vi "selection.tester.vi"() -> ()   [LabVIEW 2024]
uses:
  selection_dropdown/Typedefs/Selection Dropdown--cluster.ctl
  selection_dropdown/selection_dropdown.lvclass
  comic_manager/manager_daemon/type_defs/sub-map--map.ctl
  comic_manager/manager_daemon/type_defs/SubData--cluster.ctl
  <vilib>/addons/_JKI Toolkits/State Machine/_JKI_lib_State_Machine.llb/Select State(s)_err__jki_lib_state_machine.vi
  <vilib>/addons/_JKI Toolkits/State Machine/_JKI_lib_State_Machine.llb/Periodic Trigger__ogtk__JKI-SM__jki_lib_state_machine.vi
  comic_manager/manager_daemon/manager_daemon.lvclass
panel:
  in  "Path":path=path "D:/comics/data/key_maps/chars.bin"
  in  "Exit":bool
  in  "selection dropdown":T1
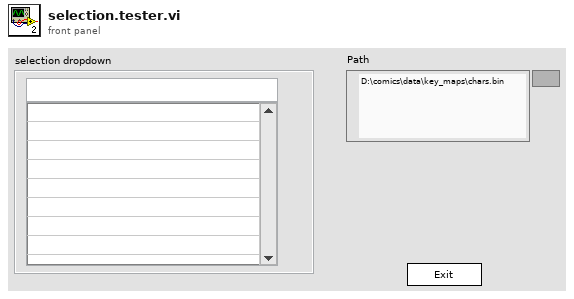
[diagram p1: front panel]
types:
  T1 = typedef "selection_dropdown.lvclass/Selection Dropdown--cluster.ctl" = cluster{"delete":bool, "available":i32, "list":i32, "cancel":bool, "selection":string, "delete all":bool}
  T2 = enum32{"Invalid", "Standard", "Closed", "Hidden", "Minimized", "Maximized"}
  T3 = enum32{"invalid app kind", "Development System", "Run Time System", "Student Edition", "Embedded LabVIEW", "Evaluation", "Custom"}
  T4 = typedef "manager_daemon.lvclass/sub-map--map.ctl" = map{string, T5}
  T5 = typedef "manager_daemon.lvclass/SubData--cluster.ctl" = cluster{"id":i32, "issues":set{i32}}
  T6 = cluster{"Core":cluster{"Current VI Reference":refnum<vi>, "Close Panel on Exit?":bool}, "selection class":refnum<class "selection_dropdown.lvclass">}
  T7 = cluster{"Current VI Reference":refnum<vi>, "Close Panel on Exit?":bool}
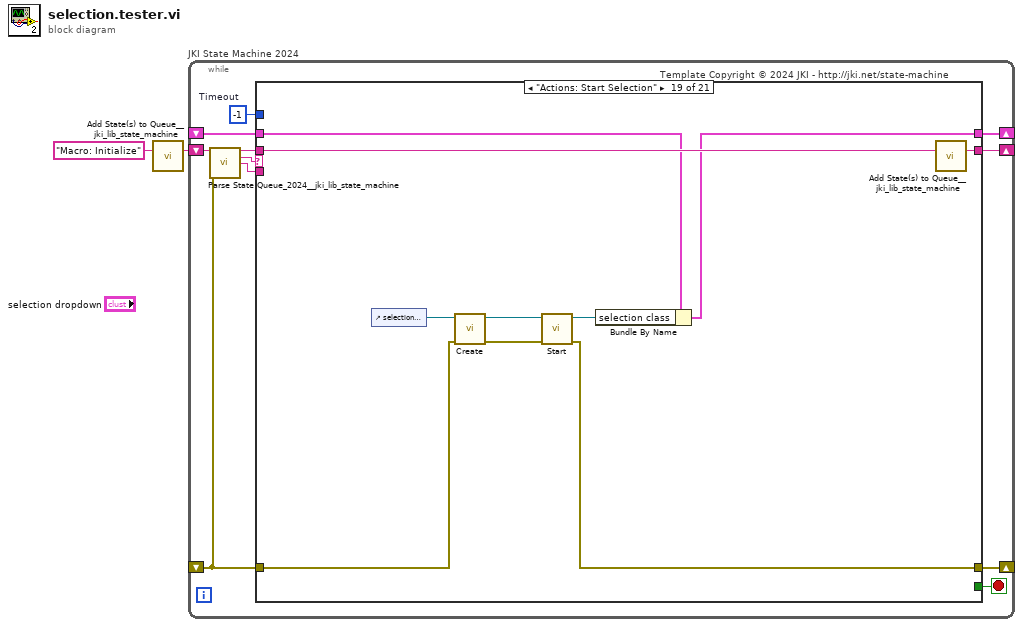
[diagram p0: block diagram]
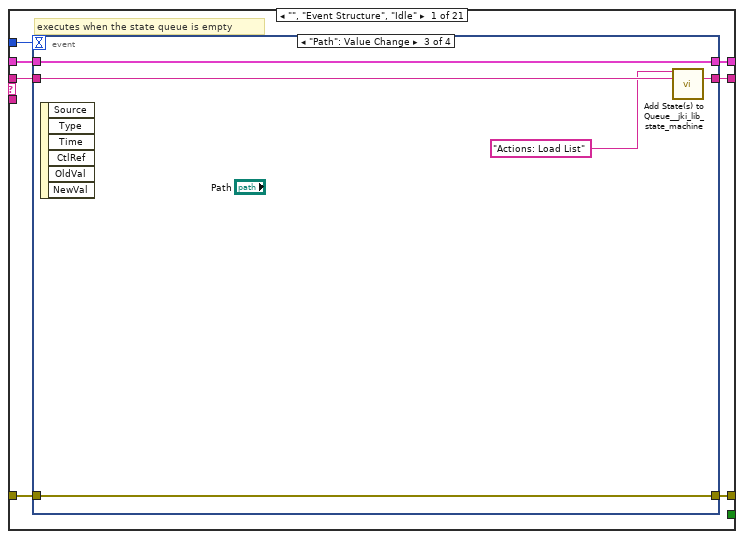
[diagram p2: hidden frame]
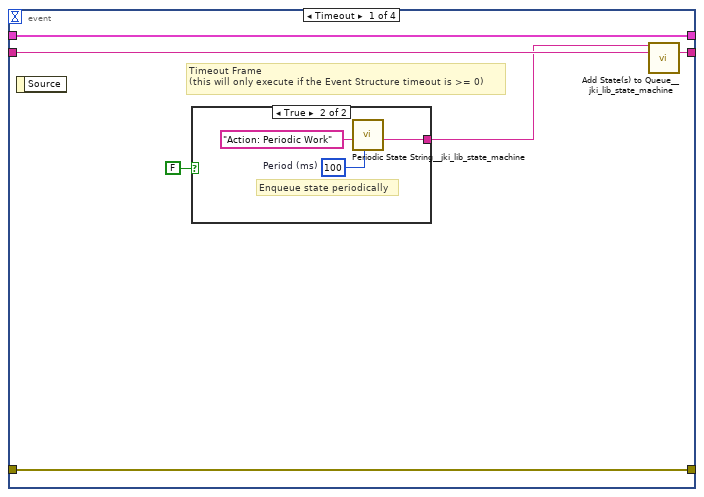
[diagram p3: hidden frame]
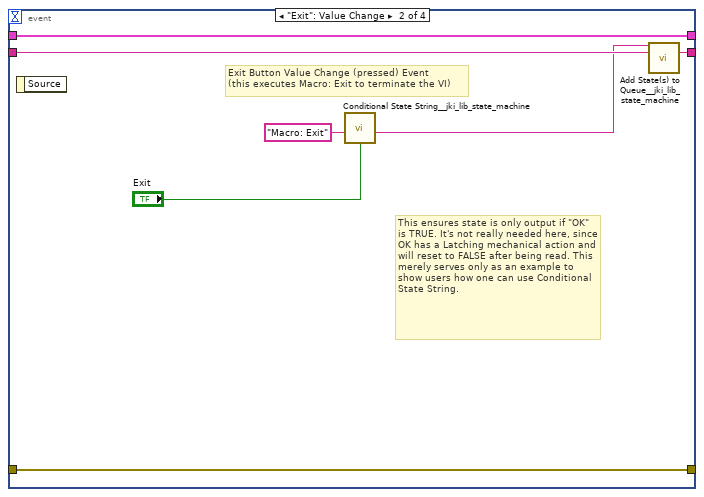
[diagram p5: hidden frame]
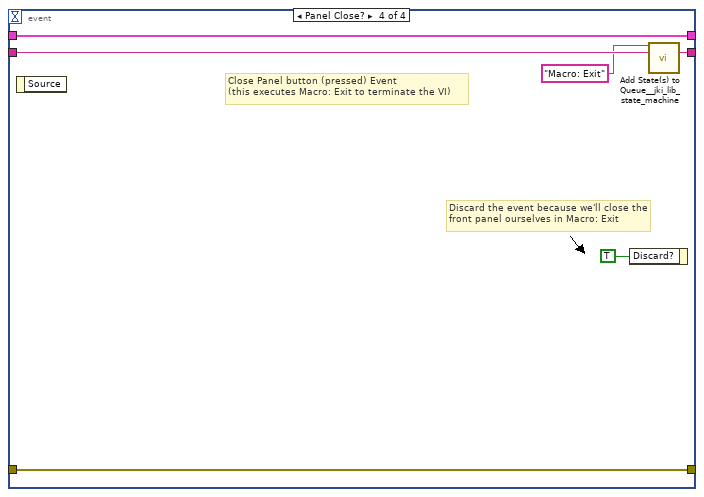
[diagram p6: hidden frame]
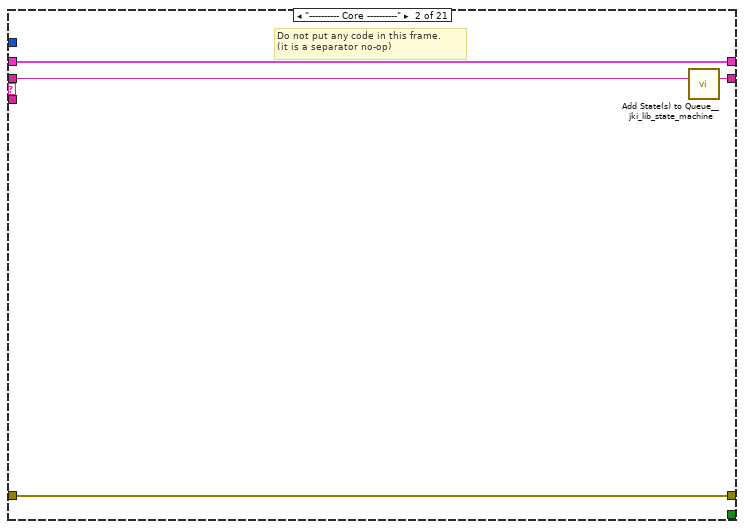
[diagram p7: hidden frame]
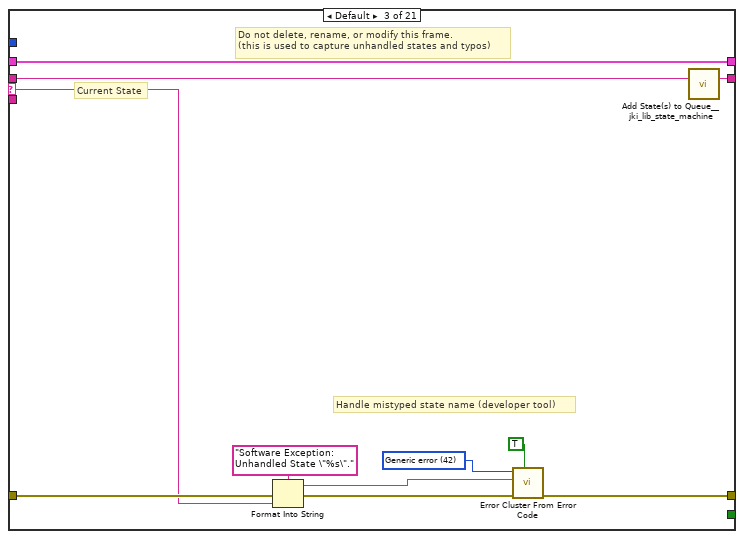
[diagram p8: hidden frame]
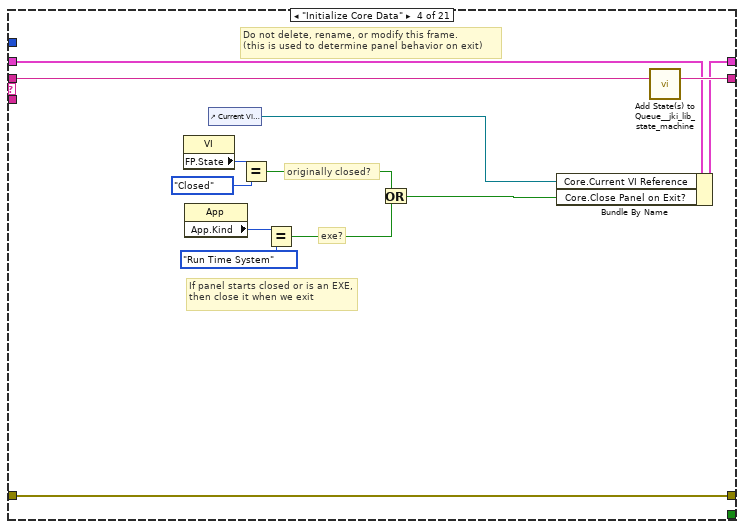
[diagram p9: hidden frame]
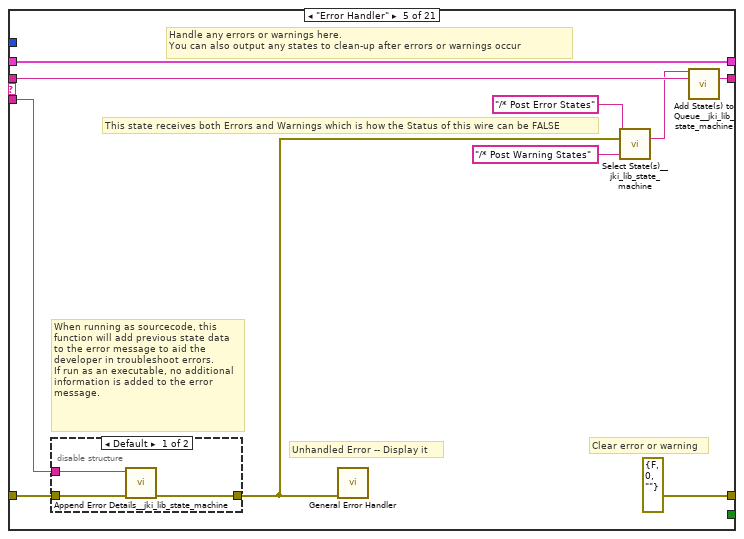
[diagram p10: hidden frame]
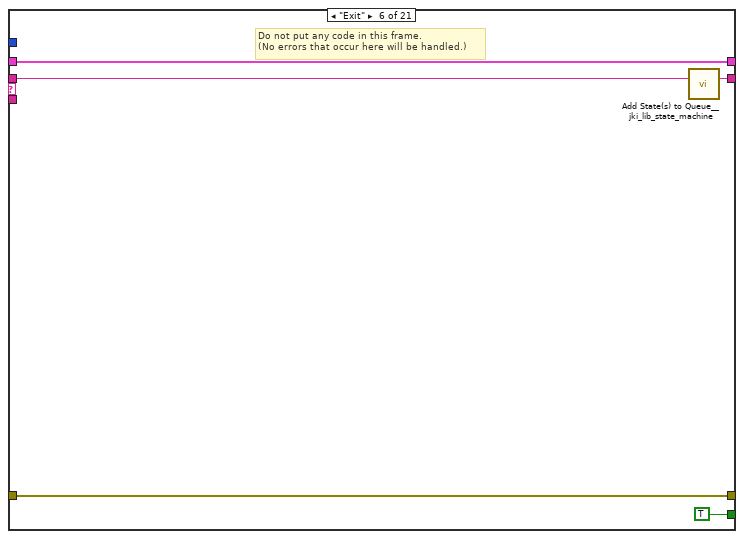
[diagram p12: hidden frame]
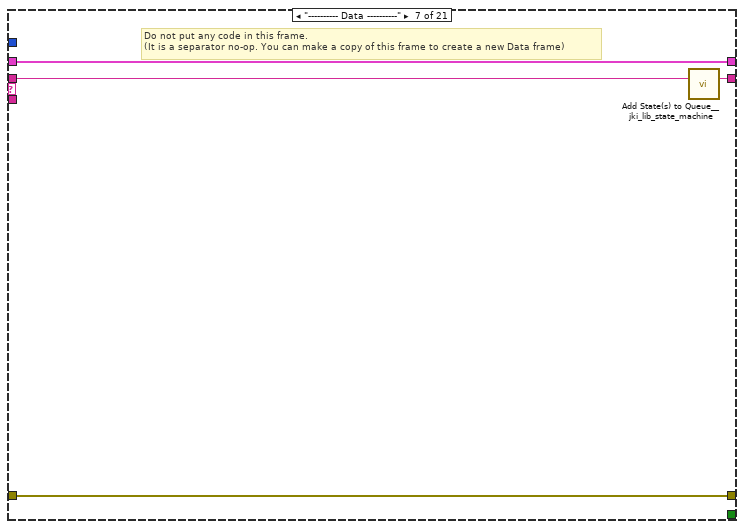
[diagram p13: hidden frame]
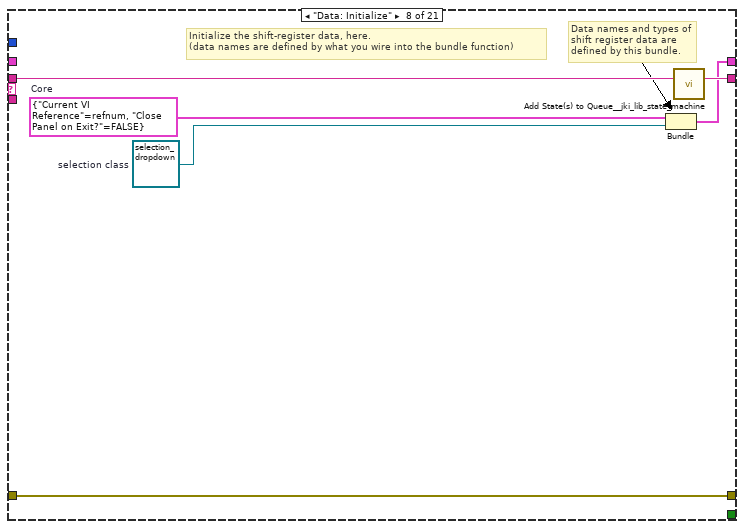
[diagram p14: hidden frame]
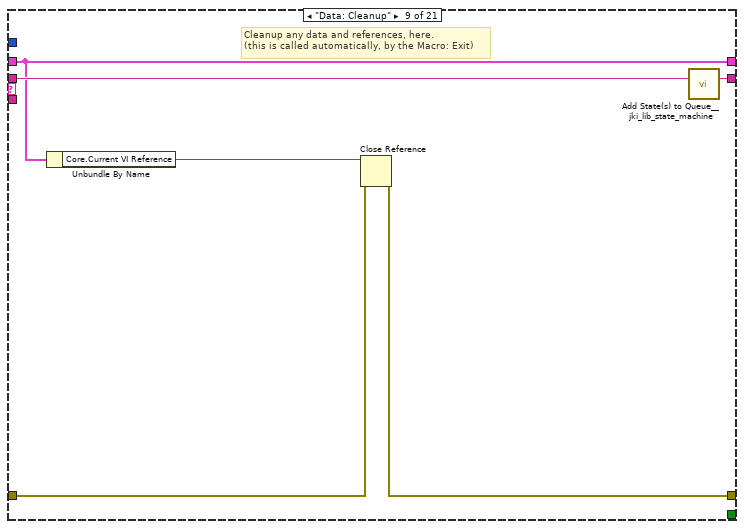
[diagram p15: hidden frame]
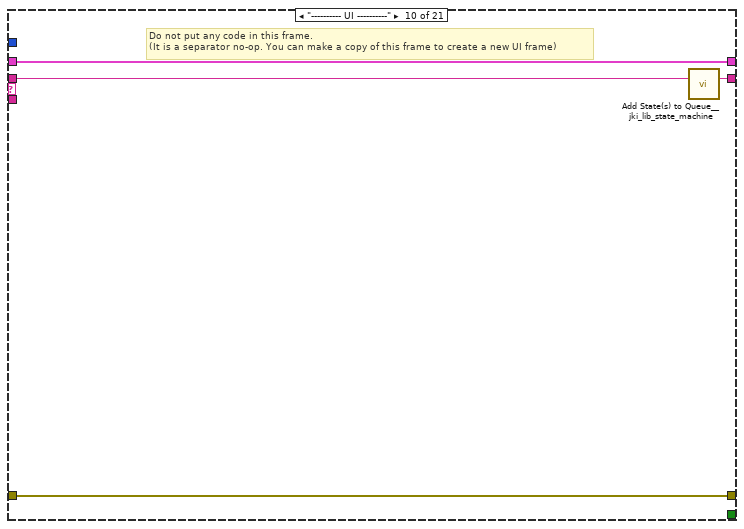
[diagram p16: hidden frame]
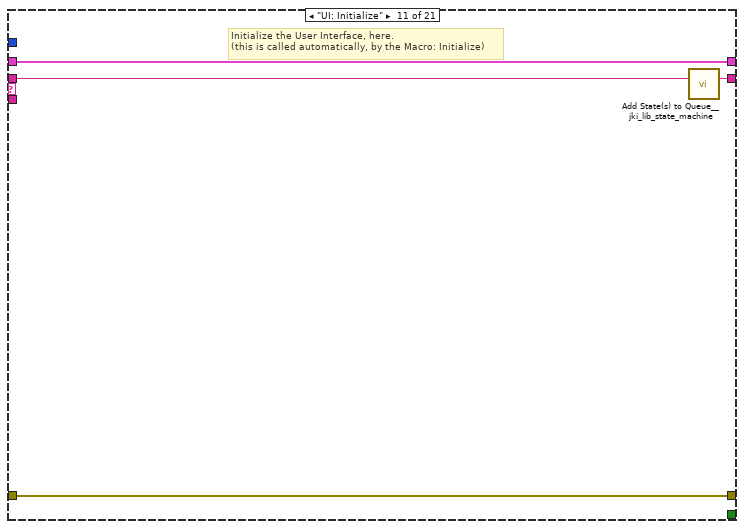
[diagram p17: hidden frame]
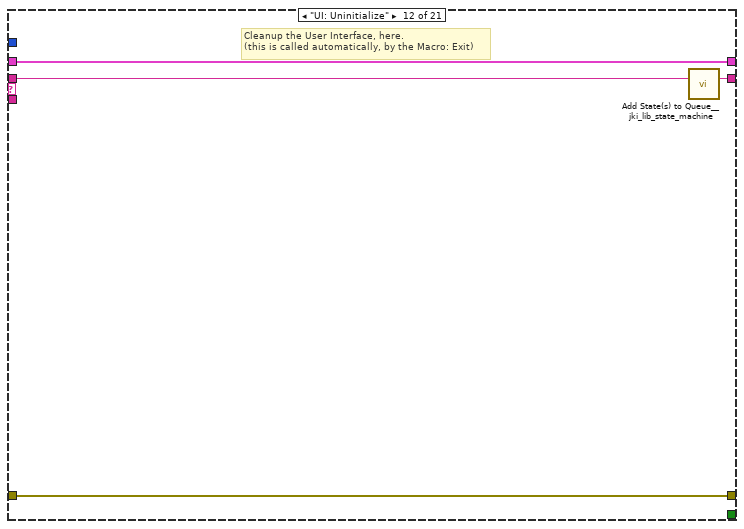
[diagram p18: hidden frame]
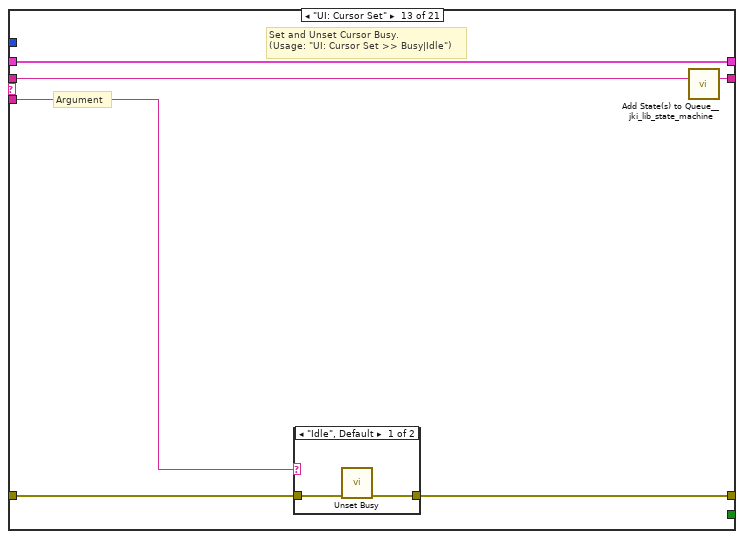
[diagram p19: hidden frame]
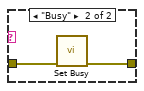
[diagram p20: hidden frame]
diagram:
  n1 = call <vilib>:"Add State(s) to Queue__jki_lib_state_machine.vi"("State(s) in (\"\")"="Macro: Initialize") -> ("States Out"=w2:string)  [unwired: 14 in]
  n2 = while "JKI State Machine 2024" {
    shift-right: [w6] -> _
    shift-left: _ -> [w5]
    shift-right: [w9] -> _
    shift-left: _ -> [w3]
    shift-right: [w8] -> _
    shift-left: w2 -> [w10]
    stop <- w7 stop-if-true
    w4 = -1  # Timeout
    # "Template Copyright © 2024 JKI - http://jki.net/state-machine"
    n3 = call <vilib>:"Parse State Queue_2024__jki_lib_state_machine.vi"("State Queue"=w10, "Error In (no error)"=w3) -> ("Remaining States"=w12:string, "Current State"=w13:string, "Arguments"=w11:string)  [unwired: 11 in]
    n4 = case shown="\"Actions: Start Selection\"" w13 {
      selector: w13 -> [_ _ w52 _ _ _ _ _ _ _ _ _ _ _ _ _ _ _ _ _ _]
      tunnel: w12 -> [w20 w51 w56 w75 w85 w94 w98 w104 w110 w114 w118 w122 w128 w139 w208 w213 w222 w226 w236 w242 w252]
      tunnel: w11 -> [_ _ _ _ w80 _ _ _ _ _ _ _ w123 w133 _ _ _ _ _ _ _]
      tunnel: w5 -> [w18 w48 w54 w68 w82 w92 w95 _ w105 w111 w116 w120 w126 w135 w205 w210 w220 w223 w230 w240 w250]
      tunnel: [w17 w49 w58 w72 errorcluster {"status"=FALSE, "code"=0, "source"=""} ("error out") w91 w96 w101 w106 w112 w115 w119 w124 w136 w206 w211 w217 w224 w231 w237 w248] -> w9
      tunnel: w3 -> [w14 w49 w57 w72 w81 w91 w96 w101 w107 w112 w115 w119 w125 w137 w206 w211 w217 w224 w234 w238 w247]
      tunnel: [w19 w50 w55 w74 w84 w93 w97 w103 w109 w113 w117 w121 w127 w138 w207 w212 w221 w225 w235 w241 w251] -> w8
      tunnel: [_ _ _ _ _ TRUE _ _ _ _ _ _ _ _ _ _ _ _ _ _ _] -> w7
      tunnel: [w16 w48 w54 w73 w82 w92 w95 w102 w105 w111 w116 w120 w126 w135 w205 w210 w220 w223 w229 w240 w250] -> w6
      tunnel: w4 -> [w15 _ _ _ _ _ _ _ _ _ _ _ _ _ _ _ _ _ _ _ _]
      frame "", "Event Structure", "Idle" {
        # "executes when the state queue is empty"
        n5 = event shown="[2] \"Path\": Value Change" {
          selector: _ -> [_ _ _ _]
          dyn-events: _ -> [_ _ _ _]
          timeout: w15 -> [_ _ _ _]
          tunnel: w20 -> [w26 w36 w41 w47]
          tunnel: [w25 w35 w40 w46] -> w19
          tunnel: w18 -> [w23 w33 w38 w44]
          tunnel: [w24 w34 w39 w45] -> w17
          tunnel: w14 -> [w24 w34 w39 w45]
          tunnel: [w23 w33 w38 w44] -> w16
          event Timeout {
            # "Timeout Frame\n(this will only execute if the Event Structure timeout is >= 0)"
            n6 = event-data() -> ()  [unwired: 1 in, 1 out]
            n7 = case shown="True" FALSE {
              tunnel: [_ w29] -> w22
              frame False {
              }
              frame True {
                w27 = u32 100  # Period (ms)
                # "Enqueue state periodically"
                n8 = call <vilib>:"Periodic State String__jki_lib_state_machine.vi"("Period (ms)"=w27, "State"="Action: Periodic Work") -> ("State Out"=w29:string)  [unwired: 9 in]
              }
            }
            n9 = call <vilib>:"Add State(s) to Queue__jki_lib_state_machine.vi"("State(s) in Front (\"\")"=w22, "State(s) in (\"\")"=w26) -> ("States Out"=w25:string)  [unwired: 13 in]
          }
          event "Exit": Value Change {
            # "This ensures state is only output if \"OK\" is TRUE. It's not really needed here, since OK has a Latching mechanical action and will reset to FALSE after being read. This merely serves only as an example to show users how one can use Conditional State String."
            # "Exit Button Value Change (pressed) Event\n(this executes Macro: Exit to terminate the VI)"
            n10 = event-data() -> ()  [unwired: 1 in, 1 out]
            n11 = call <vilib>:"Conditional State String__jki_lib_state_machine.vi"("Do State(s)?"="Exit", "State"="Macro: Exit") -> ("State Out"=w30:string)  [unwired: 7 in]
            n12 = call <vilib>:"Add State(s) to Queue__jki_lib_state_machine.vi"("State(s) in Front (\"\")"=w30, "State(s) in (\"\")"=w36) -> ("States Out"=w35:string)  [unwired: 13 in]
          }
          event "Path": Value Change {
            n13 = event-data() -> ()  [unwired: 1 in, 6 out]
            n14 = call <vilib>:"Add State(s) to Queue__jki_lib_state_machine.vi"("State(s) in Front (\"\")"="Actions: Load List", "State(s) in (\"\")"=w41) -> ("States Out"=w40:string)  [unwired: 13 in]
          }
          event Panel Close? {
            # "Discard the event because we'll close the front panel ourselves in Macro: Exit"
            # "Close Panel button (pressed) Event\n(this executes Macro: Exit to terminate the VI)"
            n15 = event-data() -> ()  [unwired: 1 in, 1 out]
            n16 = event-data("Discard?"=TRUE) -> ()  [unwired: 1 in, 1 out]
            n17 = call <vilib>:"Add State(s) to Queue__jki_lib_state_machine.vi"("State(s) in Front (\"\")"="Macro: Exit", "State(s) in (\"\")"=w47) -> ("States Out"=w46:string)  [unwired: 13 in]
          }
        }
      }
      frame "---------- Core ----------" {
        # "Do not put any code in this frame.\n(it is a separator no-op)"
        n18 = call <vilib>:"Add State(s) to Queue__jki_lib_state_machine.vi"("State(s) in (\"\")"=w51) -> ("States Out"=w50:string)  [unwired: 14 in]
      }
      frame Default {
        w61 = 42 items=["No error", "Argument error", "Memory is full", "Out of zone", "End of file", "File already open", "Generic file I/O error", "File not found", "File permission error", "Disk is full", "Duplicate path", "Too many files open", "System feature not enabled", "Resource file not found", "Cannot add resource", "Resource not found", "Image not found", "Image memory error", "Pen does not exist", "Config type invalid", "Config token not found", "Config parse error", "Config memory error", "Bad external code format", "Bad external code offset", "External code not present", "Null window", "Destroy window error", "Null menu", "Print aborted", "Bad print record", "Print driver error", "Windows error during printing", "Memory error during printing", "Print dialog error", "Generic print error", "Invalid device refnum", "Device not found", "Device parameter error", "Device unit error", "Cannot open device", "Device call aborted", "Generic error", "Cancelled by user", "Object ID too low", "Object ID too high", "Object not in heap", "Unknown heap", "Unknown object (invalid DefProc)", "Unknown object (DefProc not in table)", "Message out of range", "Invalid (null) method", "Unknown message", "Manager call not supported", "Bad address", "Network operation in progress", "Network operation timed out", "Connection is busy", "Network attribute not supported", "Network error", "Address in use", "System out of memory", "Connection aborted", "Connection refused", "Not connected", "Already connected", "Connection closed", "Initialization error (interapplication manager)", "Bad occurrence", "Wait on unbound occurrence handler", "Occurrence queue overflow", "Datalog type conflict", "Unused", "Unrecognized type (interapplication manager)", "Memory corrupt", "Failed to make temporary DLL", "Old CIN version", "Drag socket not found", "Failed to load drop-object", "Failed to register OLE object", "Failed to release OLE object", "Format specifier type mismatch", "Unknown format specifier", "Too few format specifiers", "Too many format specifiers", "Scan failed", "Newer CIN version", "Error converting to variant", "Runtime menu error", "Password tampered", "Variant attribute not found", "Incompatible variant data type", "Event data is not available", "Event Store is not present", "Occurrence is not found", "Event Queue is not created", "Event info is not available", "Refnum passed is NULL", "Error retrieving Class GUID", "Error retrieving CoClass GUID", "Error retrieving TypeLib GUID.", "Bad built application magic bytes.", "Specific driver is different from the specific driver associated with the Logical Name.", "There is no session opened to the class driver.", "Max Error", "MAX - Error with config objects", "MAX - Error loading configuration", "MAX - Group not supported"]
        # "Current State"
        # "Do not delete, rename, or modify this frame.\n(this is used to capture unhandled states and typos)"
        # "Handle mistyped state name (developer tool)"
        n19 = Format Into String(format string="Software Exception: Unhandled State \"%s\"." ("message"), error in=w57, w52) -> (resulting string=w60:string, error out=w59:errorcluster)  [unwired: 1 in]
        n20 = call <vilib>:"Error Cluster From Error Code.vi"("show call chain? (False)"=TRUE, "error in (no error)"=w59, "error message (\"\")"=w60, "error code (0)"=w61) -> ("error out"=w58:errorcluster)  [unwired: 5 in]
        n21 = call <vilib>:"Add State(s) to Queue__jki_lib_state_machine.vi"("State(s) in (\"\")"=w56) -> ("States Out"=w55:string)  [unwired: 14 in]
      }
      frame "Initialize Core Data" {
        # "Do not delete, rename, or modify this frame.\n(this is used to determine panel behavior on exit)"
        # "originally closed?"
        # "exe?"
        # "If panel starts closed or is an EXE, then close it when we exit"
        n22 = property class="VI"() -> ("FP.State"=w65:T2)  [unwired: 2 in, 2 out]
        n23 = property class="App"() -> ("App.Kind"=w71:T3)  [unwired: 2 in, 2 out]
        n24 = control-ref of="Current VI Reference"() -> (w66:refnum<vi>)
        n25 = Equal?(x=w65, y=T2."Closed" ("Front Panel Window:State")) -> (x = y?=w63:bool)
        n26 = Equal?(x=w71, y=T3."Run Time System" ("Application:Kind")) -> (x = y?=w69:bool)
        n27 = Or(x=w63, y=w69) -> (x .or. y?=w67:bool)
        n28 = Bundle By Name(cluster=w68, "Core.Current VI Reference"=w66, "Core.Close Panel on Exit?"=w67) -> (w73:T6)
        n29 = call <vilib>:"Add State(s) to Queue__jki_lib_state_machine.vi"("State(s) in (\"\")"=w75) -> ("States Out"=w74:string)  [unwired: 14 in]
      }
      frame "Error Handler" {
        # "When running as sourcecode, this function will add previous state data to the error message to aid the developer in troubleshoot errors.\nIf run as an executable, no additional information is added to the error message."
        # "This state receives both Errors and Warnings which is how the Status of this wire can be FALSE"
        # "Unhandled Error -- Display it"
        # "Handle any errors or warnings here.\nYou can also output any states to clean-up after errors or warnings occur"
        # "Clear error or warning"
        n30 = disable-structure shown="Default" {
          disable-tunnel: w81 -> [w88 w89]
          disable-tunnel: w80 -> [w87 _]
          disable-tunnel: [w86 w89] -> w79
          frame condition #0 (active) {
            n31 = call <vilib>:"Append Error Details__jki_lib_state_machine.vi"("error in (no error)"=w88, "Previous State and Argument(s)"=w87) -> ("error out"=w86:errorcluster)  [unwired: 9 in]
          }
          frame condition #1 {
          }
        }
        n32 = call <vilib>:"General Error Handler.vi"("error in (no error)"=w79) -> ()  [unwired: 10 in, 5 out]
        n33 = call-poly <vilib>:"Select State(s)__jki_lib_state_machine.vi"("State(s) if True (\"\")"="/* Post Error States", "Select"=w79, "State(s) if False (\"\")"="/* Post Warning States") -> ("States Out"=w77:string)  [unwired: 12 in]
        n34 = call <vilib>:"Add State(s) to Queue__jki_lib_state_machine.vi"("State(s) in Front (\"\")"=w77, "State(s) in (\"\")"=w85) -> ("States Out"=w84:string)  [unwired: 13 in]
      }
      frame "Exit" {
        # "Do not put any code in this frame.\n(No errors that occur here will be handled.)"
        n35 = call <vilib>:"Add State(s) to Queue__jki_lib_state_machine.vi"("State(s) in (\"\")"=w94) -> ("States Out"=w93:string)  [unwired: 14 in]
      }
      frame "---------- Data ----------" {
        # "Do not put any code in this frame.\n(It is a separator no-op. You can make a copy of this frame to create a new Data frame)"
        n36 = call <vilib>:"Add State(s) to Queue__jki_lib_state_machine.vi"("State(s) in (\"\")"=w98) -> ("States Out"=w97:string)  [unwired: 14 in]
      }
      frame "Data: Initialize" {
        w99 = refnum<class "selection_dropdown.lvclass"> refnum  # selection class
        w100 = T7 {"Current VI Reference"=refnum, "Close Panel on Exit?"=FALSE}  # Core
        # "Data names and types of shift register data are defined by this bundle."
        # "Initialize the shift-register data, here.\n(data names are defined by what you wire into the bundle function)"
        n37 = Bundle("Core"=w100, "selection class"=w99) -> (w102:T6)  [unwired: 1 in]
        n38 = call <vilib>:"Add State(s) to Queue__jki_lib_state_machine.vi"("State(s) in (\"\")"=w104) -> ("States Out"=w103:string)  [unwired: 14 in]
      }
      frame "Data: Cleanup" {
        # "Cleanup any data and references, here.\n(this is called automatically, by the Macro: Exit)"
        n39 = Unbundle By Name(w105) -> ("Core.Current VI Reference"=w108:refnum<vi>)
        n40 = Close Reference(reference=w108, error in (no error)=w107) -> (error out=w106:errorcluster)
        n41 = call <vilib>:"Add State(s) to Queue__jki_lib_state_machine.vi"("State(s) in (\"\")"=w110) -> ("States Out"=w109:string)  [unwired: 14 in]
      }
      frame "---------- UI ----------" {
        # "Do not put any code in this frame.\n(It is a separator no-op. You can make a copy of this frame to create a new UI frame)"
        n42 = call <vilib>:"Add State(s) to Queue__jki_lib_state_machine.vi"("State(s) in (\"\")"=w114) -> ("States Out"=w113:string)  [unwired: 14 in]
      }
      frame "UI: Initialize" {
        # "Initialize the User Interface, here.\n(this is called automatically, by the Macro: Initialize)"
        n43 = call <vilib>:"Add State(s) to Queue__jki_lib_state_machine.vi"("State(s) in (\"\")"=w118) -> ("States Out"=w117:string)  [unwired: 14 in]
      }
      frame "UI: Uninitialize" {
        # "Cleanup the User Interface, here.\n(this is called automatically, by the Macro: Exit)"
        n44 = call <vilib>:"Add State(s) to Queue__jki_lib_state_machine.vi"("State(s) in (\"\")"=w122) -> ("States Out"=w121:string)  [unwired: 14 in]
      }
      frame "UI: Cursor Set" {
        # "Argument"
        # "Set and Unset Cursor Busy.\n(Usage: \"UI: Cursor Set >> Busy|Idle\")"
        n45 = case shown="\"Idle\", Default" w123 {
          tunnel: w125 -> [w130 w132]
          tunnel: [w129 w131] -> w124
          frame "Idle", Default {
            n46 = call <vilib>:"Unset Busy.vi"("error in (no error)"=w130) -> ("error out"=w129:errorcluster)  [unwired: 10 in]
          }
          frame "Busy" {
            n47 = call <vilib>:"Set Busy.vi"("error in (no error)"=w132) -> ("error out"=w131:errorcluster)  [unwired: 9 in, 1 out]
          }
        }
        n48 = call <vilib>:"Add State(s) to Queue__jki_lib_state_machine.vi"("State(s) in (\"\")"=w128) -> ("States Out"=w127:string)  [unwired: 14 in]
      }
      frame "UI: Front Panel State" {
        # "Argument"
        # "Set Front Panel Open or Closed\n(Usage: \"UI: Front Panel State >> Open|Close\")"
        n49 = Unbundle By Name(w135) -> ("Core.Current VI Reference"=w134:refnum<vi>)
        n50 = case shown="\"Minimize\", \"Minimized\"" w133 {
          tunnel: w137 -> [w145 w160 w171 w184 w197]
          tunnel: [w147 w161 w173 w186 w199] -> w136
          tunnel: w134 -> [w146 w158 w172 w185 w198]
          frame "Open", "Standard", Default {
            w140 = T2."Standard" ("State")
            n51 = property class="VI"(reference=w146, error in=w145) -> (reference out=w143:refnum<vi>, error out=w144:errorcluster, "FP.State"=w142:T2)
            n52 = Not Equal?(x=w142, y=w140) -> (x != y?=w141:bool)
            n53 = case shown="True" w141 {
              tunnel: [w151 w153] -> w147
              tunnel: w144 -> [w150 w153]
              tunnel: w143 -> [w149 _]
              tunnel: w140 -> [w148 _]
              frame True {
                n54 = invoke class="VI" method="FP.Open"(reference=w149, error in=w150, "Activate"=TRUE, "State"=w148) -> (error out=w151:errorcluster)  [unwired: 1 in, 4 out]
              }
              frame False {
              }
            }
          }
          frame "Close", "Closed" {
            n55 = property class="VI"(reference=w158, error in=w160) -> (reference out=w157:refnum<vi>, error out=w159:errorcluster, "FP.State"=w155:T2)
            n56 = Not Equal?(x=w155, y=T2."Closed" ("Front Panel Window:State")) -> (x != y?=w154:bool)
            n57 = case shown="True" w154 {
              tunnel: [w162 w165] -> w161
              tunnel: w159 -> [w162 w164]
              tunnel: w157 -> [_ w163]
              frame False {
              }
              frame True {
                n58 = invoke class="VI" method="FP.Close"(reference=w163, error in=w164) -> (error out=w165:errorcluster)  [unwired: 1 in, 2 out]
              }
            }
          }
          frame "Hidden", "Hide" {
            w166 = T2."Hidden" ("State")
            n59 = property class="VI"(reference=w172, error in=w171) -> (reference out=w169:refnum<vi>, error out=w170:errorcluster, "FP.State"=w168:T2)
            n60 = Not Equal?(x=w168, y=w166) -> (x != y?=w167:bool)
            n61 = case shown="True" w167 {
              tunnel: [w177 w178] -> w173
              tunnel: w170 -> [w176 w178]
              tunnel: w169 -> [w175 _]
              tunnel: w166 -> [w174 _]
              frame True {
                n62 = invoke class="VI" method="FP.Open"(reference=w175, error in=w176, "State"=w174) -> (error out=w177:errorcluster)  [unwired: 2 in, 4 out]
              }
              frame False {
              }
            }
          }
          frame "Minimize", "Minimized" {
            w179 = T2."Minimized" ("State")
            n63 = property class="VI"(reference=w185, error in=w184) -> (reference out=w182:refnum<vi>, error out=w183:errorcluster, "FP.State"=w181:T2)
            n64 = Not Equal?(x=w181, y=w179) -> (x != y?=w180:bool)
            n65 = case shown="True" w180 {
              tunnel: [w190 w191] -> w186
              tunnel: w183 -> [w189 w191]
              tunnel: w182 -> [w188 _]
              tunnel: w179 -> [w187 _]
              frame True {
                n66 = invoke class="VI" method="FP.Open"(reference=w188, error in=w189, "State"=w187) -> (error out=w190:errorcluster)  [unwired: 2 in, 4 out]
              }
              frame False {
              }
            }
          }
          frame "Maximize", "Maximized" {
            w192 = T2."Maximized" ("State")
            n67 = property class="VI"(reference=w198, error in=w197) -> (reference out=w195:refnum<vi>, error out=w196:errorcluster, "FP.State"=w194:T2)
            n68 = Not Equal?(x=w194, y=w192) -> (x != y?=w193:bool)
            n69 = case shown="True" w193 {
              tunnel: [w203 w204] -> w199
              tunnel: w196 -> [w202 w204]
              tunnel: w195 -> [w201 _]
              tunnel: w192 -> [w200 _]
              frame True {
                n70 = invoke class="VI" method="FP.Open"(reference=w201, error in=w202, "State"=w200) -> (error out=w203:errorcluster)  [unwired: 2 in, 4 out]
              }
              frame False {
              }
            }
          }
        }
        n71 = call <vilib>:"Add State(s) to Queue__jki_lib_state_machine.vi"("State(s) in (\"\")"=w139) -> ("States Out"=w138:string)  [unwired: 14 in]
      }
      frame "---------- Macro ----------" {
        # "Do not put any code in this frame.\n(It is a separator no-op. You can make a copy of this frame to create a new Macro frame)"
        n72 = call <vilib>:"Add State(s) to Queue__jki_lib_state_machine.vi"("State(s) in (\"\")"=w208) -> ("States Out"=w207:string)  [unwired: 14 in]
      }
      frame "Macro: Initialize" {
        w209 = "Data: Initialize\nInitialize Core Data\nUI: Initialize\nUI: Front Panel State >> Open\nActions: Start Selection\nActions: Load List"  # Data: Initialize Initialize Core Data UI: Initialize UI: Front Panel State >> Open Actions: Start Selection Actions: Load List
        # "Initialization Macro\n(This is called once, when the VI starts)"
        n73 = call <vilib>:"Add State(s) to Queue__jki_lib_state_machine.vi"("State(s) in Front (\"\")"=w209, "State(s) in (\"\")"=w213) -> ("States Out"=w212:string)  [unwired: 13 in]
      }
      frame "Macro: Exit" {
        # "Exit Macro\n(This is called once, when the VI exits)"
        n74 = Unbundle By Name(w220) -> ("Core.Close Panel on Exit?"=w215:bool)
        n75 = call <vilib>:"Conditional State String__jki_lib_state_machine.vi"("Do State(s)?"=w215, "State"="UI: Front Panel State >> Close") -> ("State Out"=w214:string)  [unwired: 7 in]
        n76 = call <vilib>:"Add State(s) to Queue__jki_lib_state_machine.vi"("State(s) in (\"\")"=w214, "State(s) at Back (\"\")"="UI: Uninitialize\nData: Cleanup\nActions: Close Selection\nExit") -> ("States Out"=w218:string)  [unwired: 13 in]
        n77 = call <vilib>:"Add State(s) to Queue__jki_lib_state_machine.vi"("State(s) in Front (\"\")"=w218, "State(s) in (\"\")"=w222) -> ("States Out"=w221:string)  [unwired: 13 in]
      }
      frame "---------- Actions ----------" {
        # "Template Separator\n(You can make a copy of, or modify, this frame)"
        n78 = call <vilib>:"Add State(s) to Queue__jki_lib_state_machine.vi"("State(s) in (\"\")"=w226) -> ("States Out"=w225:string)  [unwired: 14 in]
      }
      frame "Actions: Start Selection" {
        n79 = control-ref of="selection dropdown"() -> (w227:refnum<vi>)
        n80 = call "Create.vi"("error in (no error)"=w234, "ref"=w227) -> ("error out"=w233:errorcluster, "selection_dropdown out"=w232:refnum<class "selection_dropdown.lvclass">)  [unwired: 8 in]
        n81 = call "Start.vi"("error in (no error)"=w233, "selection_dropdown in"=w232) -> ("error out"=w231:errorcluster, "selection_dropdown out"=w228:refnum<class "selection_dropdown.lvclass">)  [unwired: 8 in]
        n82 = Bundle By Name(cluster=w230, "selection class"=w228) -> (w229:T6)
        n83 = call <vilib>:"Add State(s) to Queue__jki_lib_state_machine.vi"("State(s) in (\"\")"=w236) -> ("States Out"=w235:string)  [unwired: 14 in]
      }
      frame "Actions: Close Selection" {
        n84 = Unbundle By Name(w240) -> ("selection class"=w239:refnum<class "selection_dropdown.lvclass">)
        n85 = call "Destroy.vi"("error in (no error)"=w238, "selection_dropdown in"=w239) -> ("error out"=w237:errorcluster)  [unwired: 8 in, 1 out]
        n86 = call <vilib>:"Add State(s) to Queue__jki_lib_state_machine.vi"("State(s) in (\"\")"=w242) -> ("States Out"=w241:string)  [unwired: 14 in]
      }
      frame "Actions: Load List" {
        n87 = Unbundle By Name(w250) -> ("selection class"=w249:refnum<class "selection_dropdown.lvclass">)
        n88 = local read "Path"() -> (w245:path)
        n89 = Read from Binary File(5:T4 {} ("char map"), 8:w247, 11:w245) -> (0:w246:errorcluster, 2:w244:T4)  [unwired: 3 in, 2 out]
        n90 = call-dynamic "Avail List.set.vi"("error in (no error)"=w246, "detail map"=w244, "selection_dropdown in"=w249) -> ("error out"=w248:errorcluster)  [unwired: 7 in, 1 out]
        n91 = call <vilib>:"Add State(s) to Queue__jki_lib_state_machine.vi"("State(s) in (\"\")"=w252) -> ("States Out"=w251:string)  [unwired: 14 in]
      }
    }
  }
